vi "test Log File Decimation Channel (Enable Logging Then Open File).vi"(8 "error in":errorcluster, 11 "TestCase in":refnum<class "Embedded Data Logger Windows System Tests.lvclass">) -> (0 "error out":errorcluster, 3 "TestCase out":refnum<class "Embedded Data Logger Windows System Tests.lvclass">)   [LabVIEW 2027, in "Embedded Data Logger Windows System Tests.lvclass"]
uses:
  Embedded Data Logger Windows System Tests.lvclass
  C:/Program Files/National Instruments/LabVIEW 2027/vi.lib/addons/_JKI Toolkits/VI Tester/TestCase.llb/TestCase.lvclass
  <vilib>/addons/_JKI Toolkits/VI Tester/TestCase.llb/TestCase.lvclass
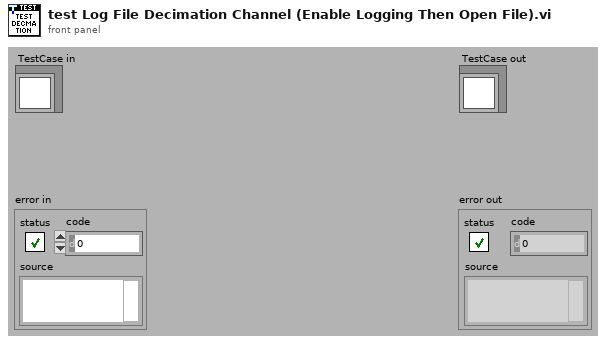
[diagram p1: front panel]
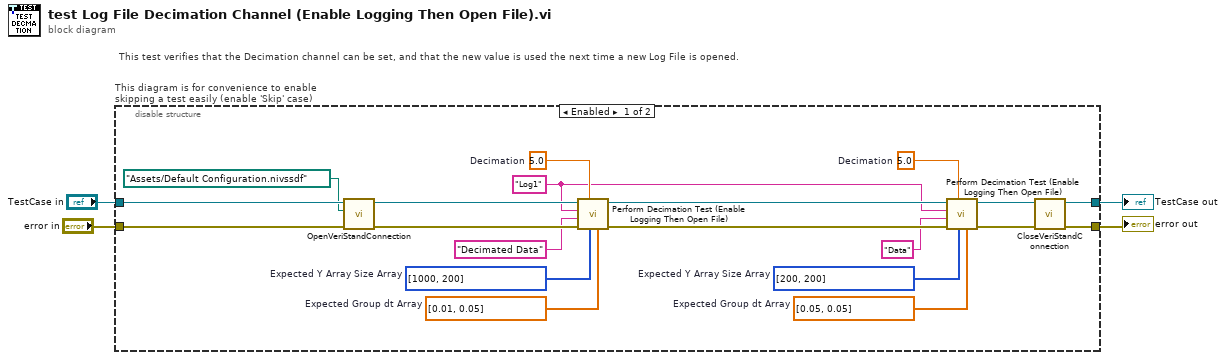
[diagram p0: block diagram]
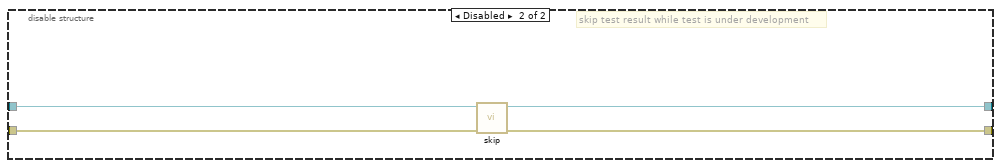
[diagram p2: hidden frame]
diagram:
  # "This test verifies that the Decimation channel can be set, and that the new value is used the next time a new Log File is opened."
  n1 = disable-structure "This diagram is for convenience to enable skipping a test easily (enable 'Skip' case)" shown="Enabled" {
    disable-tunnel: "TestCase in" -> [w23 w28]
    disable-tunnel: [w20 w26] -> w1
    disable-tunnel: [w21 w27] -> w3
    disable-tunnel: "error in" -> [w24 w25]
    frame Enabled {
      w6 = i32[] [200, 200]  # Expected Y Array Size Array
      w5 = dbl[] [0.05, 0.05]  # Expected Group dt Array
      w9 = 5.0  # Decimation
      w19 = i32[] [1000, 200]  # Expected Y Array Size Array
      w14 = dbl[] [0.01, 0.05]  # Expected Group dt Array
      w16 = 5.0  # Decimation
      w7 = "Log1" ("Embedded Data Logger File Name")
      n2 = call-dynamic "OpenVeriStandConnection.vi"("error in (no error)"=w24, "System Definition File"=path "Assets/Default Configuration.nivssdf", "VeriStand Test Case in"=w23) -> ("error out"=w17:errorcluster, "VeriStand Test Case out"=w18:refnum<class "Embedded Data Logger Windows System Tests.lvclass">)  [unwired: 6 in, 1 out]
      n3 = call "Perform Decimation Test (Enable Logging Then Open File).vi"("Expected Group dts"=w14, "Expected Y Array Sizes"=w19, "Decimation"=w16, "error in"=w17, "Embedded Data Logger Channel Group Name"="Decimated Data" ("Embedded Data Logger File Name"), "Embedded Data Logger File Name"=w7, "Embedded Data Logger Windows System Tests in"=w18) -> ("error out"=w11:errorcluster, "Embedded Data Logger Windows System Tests out"=w13:refnum<class "Embedded Data Logger Windows System Tests.lvclass">)  [unwired: 3 in]
      n4 = call "Perform Decimation Test (Enable Logging Then Open File).vi"("Expected Group dts"=w5, "Expected Y Array Sizes"=w6, "Decimation"=w9, "error in"=w11, "Embedded Data Logger Channel Group Name"="Data" ("Embedded Data Logger File Name"), "Embedded Data Logger File Name"=w7, "Embedded Data Logger Windows System Tests in"=w13) -> ("error out"=w10:errorcluster, "Embedded Data Logger Windows System Tests out"=w12:refnum<class "Embedded Data Logger Windows System Tests.lvclass">)  [unwired: 3 in]
      n5 = call-dynamic "CloseVeriStandConnection.vi"("error in (no error)"=w10, "VeriStand Test Case in"=w12) -> ("error out"=w21:errorcluster, "VeriStand Test Case out"=w20:refnum<class "Embedded Data Logger Windows System Tests.lvclass">)  [unwired: 8 in]
    }
    frame Disabled {
      # "skip test result while test is under development"
      n6 = call <vilib>:"skip.vi"("error in (no error)"=w25, "TestCase in"=w28) -> ("error out"=w27:errorcluster, "TestCase out"=w26:refnum<class "Embedded Data Logger Windows System Tests.lvclass">)  [unwired: 8 in]
    }
  }
  "error out" <- w3
  "TestCase out" <- w1
